vi "SetAttributeViBoolean_CP_Monitor_PS_Waveform.vi"(7 "AttributeValue (Off)":bool, 8 "error in (no error)":errorcluster {"code" format="%.0x"}, 9 "AttributeID":u32(ring)=1150049 items=["CHANNELPOWER_AVERAGE_ENABLED"=1150049, "CHANNELPOWER_DETECTOR_AUTO"=1150109, "CHANNELPOWER_DISPLAY_BAR_GRAPH_ENABLED"=1190232, "CHANNELPOWER_DISPLAY_WINDOWY_AUTO_SCALE_ENABLED"=1190236, "CHANNELPOWER_FILTER_ENABLED"=1190238, "CHANNELPOWER_FREQUENCY_PHASE_NOISE_OPTION_AUTO_ENABLED"=1190659, "CHANNELPOWER_IF_GAIN_AUTO_ENABLED"=1150041, "CHANNELPOWER_IF_GAIN"=1150038, "CHANNELPOWER_MARKER_COUPLE_ENABLED"=1190668, "CHANNELPOWER_MARKER_ENABLED"=1190253, "CHANNELPOWER_POWER_LIMIT_ENABLED"=1191767, "CHANNELPOWER_PSD_LIMIT_ENABLED"=1191690, "CHANNELPOWER_SWEEPCOUPLING_RESOLUTION_BANDWIDTH_AUTO_ENABLED"=1190257, "CHANNELPOWER_SWEEPCOUPLING_SWEEP_TIME_AUTO_ENABLED"=1190260, "CHANNELPOWER_SWEEPCOUPLING_VIDEO_BANDWIDTH_AUTO_ENABLED"=1190263, "CONTINUOUS_PEAK_SEARCH_ENABLED"=1191709, "MONITOR_AVERAGE_ENABLED"=1190349, "MONITOR_DISPLAY_AUTO_WINDOWY_SCALE_ENABLED"=1190354, "MONITOR_FREQUENCY_SPAN_RESOLUTION_BANDWIDTH_RATIO_AUTO_ENABLED"=1190345, "MONITOR_MARKER_COUPLE_ENABLED"=1190371, "MONITOR_MARKER_ENABLED"=1191684, "MONITOR_SWEEPCOUPLING_RESOLUTION_BANDWIDTH_AUTO_ENABLED"=1190361, "MONITOR_SWEEPCOUPLING_SWEEP_TIME_AUTO_ENABLED"=1190364, "MONITOR_SWEEPCOUPLING_VIDEO_BANDWIDTH_AUTO_ENABLED"=1190366, "MONITOR_SWEEPCOUPLING_VIDEO_BANDWIDTH_RATIO_AUTO_ENABLED"=1150113, "MONITOR_TRACE_DETECTOR_TYPE_AUTO_ENABLED"=1190347, "MONITOR_TRACE_DISPLAY_ENABLED"=1190009, "MONITOR_TRACE_UPDATE_ENABLED"=1190040, "POWER_STATISTICS_DISPLAY_GAUSSIAN_LINE_ENABLED"=1190431, "POWER_STATISTICS_DISPLAY_REFERENCE_TRACE_ENABLED"=1190432, "POWER_STATISTICS_IF_GAIN_AUTO_ENABLED"=1190419, "POWER_STATISTICS_IF_GAIN"=1190418, "POWER_STATISTICS_MARKER_COUPLE_ENABLED"=1190426, "POWER_STATISTICS_MARKER_ENABLED"=1191685, "WAVEFORM_ADC_DITHER_AUTO_ENABLED"=1190536, "WAVEFORM_ADC_DITHER_ENABLED"=1190535, "WAVEFORM_AVERAGE_ENABLED"=1190538, "WAVEFORM_AVERAGE_TIME_AVERAGE_COUNT_AUTO_ENABLED"=1191503, "WAVEFORM_DISPLAY_IQWAVEFORM_VIEW_WINDOWX_AUTO_SCALE_ENABLED"=1191577, "WAVEFORM_DISPLAY_IQWAVEFORM_VIEW_WINDOWY_AUTO_SCALE_ENABLED"=1191581, "WAVEFORM_DISPLAY_WINDOWX_AUTO_SCALE_ENABLED"=1190547, "WAVEFORM_DISPLAY_WINDOWY_AUTO_SCALE_ENABLED"=1190550, "WAVEFORM_FILTER_BANDWIDTH_AUTO_ENABLED"=1191499, "WAVEFORM_FREQUENCY_SYNTHESIS_STATE_AUTO_ENABLED"=1191507, "WAVEFORM_IF_GAIN_AUTO_ENABLED"=1190532, "WAVEFORM_MARKER_COUPLE_ENABLED"=1190554, "WAVEFORM_MARKER_ENABLED"=1190556], 10 "RepCapIdentifier":string, 11 "instrument handle":refnum<k15>) -> (0 "error out":errorcluster {"code" format="%.0x"}, 3 "instrument handle out":refnum<k15>)   [LabVIEW 2021, in "Keysight XSAnVMA.lvlib"]
doc: "Sets Boolean Attribute from instrumrnt driver.\nThe following attributes are supported:\n\nCHANNELPOWER_AVERAGE_ENABLED\nCHANNELPOWER_DETECTOR_AUTO\nCHANNELPOWER_DISPLAY_BAR_GRAPH_ENABLED\nCHANNELPOWER_DISPLAY_WINDOWY_AUTO_SCALE_ENABLED\nCHANNELPOWER_FILTER_ENABLED\nCHANNELPOWER_FREQUENCY_PHASE_NOISE_OPTION_AUTO_ENABLED\nCHANNELPOWER_IF_GAIN_AUTO_ENABLED\nCHANNELPOWER_IF_GAIN\nCHANNELPOWER_MARKER_COUPLE_ENABLED\nCHANNELPOWER_MARKER_ENABLED\nCHANNELPOWER_POWER_LIMIT_ENABLED\nCHANNELPOWER_PSD_LIMIT_ENABLED\nCHANNELPOWER_SWEEPCOUPLING_RESOLUTION_BANDWIDTH_AUTO_ENABLED\nCHANNELPOWER_SWEEPCOUPLING_SWEEP_TIME_AUTO_ENABLED\nCHANNELPOWER_SWEEPCOUPLING_VIDEO_BANDWIDTH_AUTO_ENABLED\nCONTINUOUS_PEAK_SEARCH_ENABLED\nMONITOR_AVERAGE_ENABLED\nMONITOR_DISPLAY_AUTO_WINDOWY_SCALE_ENABLED\nMONITOR_FREQUENCY_SPAN_RESOLUTION_BANDWIDTH_RATIO_AUTO_ENABLED\nMONITOR_MARKER_COUPLE_ENABLED\nMONITOR_MARKER_ENABLED\nMONITOR_SWEEPCOUPLING_RESOLUTION_BANDWIDTH_AUTO_ENABLED\nMONITOR_SWEEPCOUPLING_SWEEP_TIME_AUTO_ENABLED\nMONITOR_SWEEPCOUPLING_VIDEO_BANDWIDTH_AUTO_ENABLED\nMONITOR_SWEEPCOUPLING_VIDEO_BANDWIDTH_RATIO_AUTO_ENABLED\nMONITOR_TRACE_DETECTOR_TYPE_AUTO_ENABLED\nMONITOR_TRACE_DISPLAY_ENABLED\nMONITOR_TRACE_UPDATE_ENABLED\nPOWER_STATISTICS_DISPLAY_GAUSSIAN_LINE_ENABLED\nPOWER_STATISTICS_DISPLAY_REFERENCE_TRACE_ENABLED\nPOWER_STATISTICS_IF_GAIN_AUTO_ENABLED\nPOWER_STATISTICS_IF_GAIN\nPOWER_STATISTICS_MARKER_COUPLE_ENABLED\nPOWER_STATISTICS_MARKER_ENABLED\nWAVEFORM_ADC_DITHER_AUTO_ENABLED\nWAVEFORM_ADC_DITHER_ENABLED\nWAVEFORM_AVERAGE_ENABLED\nWAVEFORM_AVERAGE_TIME_AVERAGE_COUNT_AUTO_ENABLED\nWAVEFORM_DISPLAY_IQWAVEFORM_VIEW_WINDOWX_AUTO_SCALE_ENABLED\nWAVEFORM_DISPLAY_IQWAVEFORM_VIEW_WINDOWY_AUTO_SCALE_ENABLED\nWAVEFORM_DISPLAY_WINDOWX_AUTO_SCALE_ENABLED\nWAVEFORM_DISPLAY_WINDOWY_AUTO_SCALE_ENABLED\nWAVEFORM_FILTER_BANDWIDTH_AUTO_ENABLED\nWAVEFORM_FREQUENCY_SYNTHESIS_STATE_AUTO_ENABLED\nWAVEFORM_IF_GAIN_AUTO_ENABLED\nWAVEFORM_MARKER_COUPLE_ENABLED\nWAVEFORM_MARKER_ENABLED"
uses:
  <instrlib>/Keysight XSAnVMA/Keysight XSAnVMA.lvlib
  KtXSAnVMA_64.dll
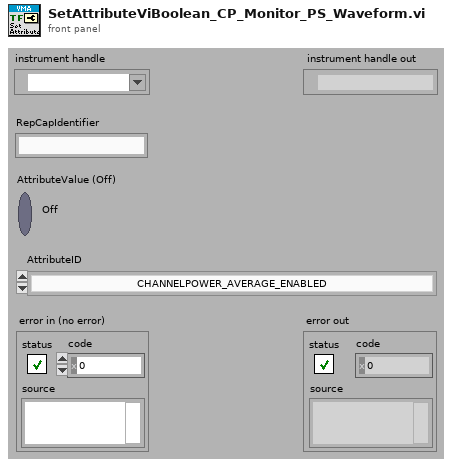
[diagram p1: front panel]
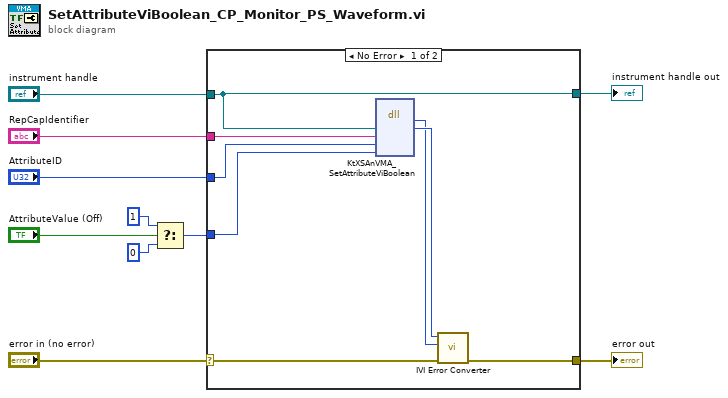
[diagram p0: block diagram]
diagram:
  n1 = Select(t=u16 1, s="AttributeValue (Off)", f=u16 0) -> (s? t:f=w3:u16)
  n2 = case shown="No Error" "error in (no error)" {
    selector: "error in (no error)" -> [w16 w20]
    tunnel: [w15 w20] -> w10
    tunnel: "instrument handle" -> [w11 w19]
    tunnel: "RepCapIdentifier" -> [w14 _]
    tunnel: "AttributeID" -> [w13 _]
    tunnel: w3 -> [w12 _]
    tunnel: [w11 w19] -> w1
    frame No Error {
      n3 = dll-call lib="KtXSAnVMA**.dll" fn="KtXSAnVMA_SetAttributeViBoolean"("Vi"=w11, "RepCapIdentifier"=w14, "AttributeID"=w13, "AttributeValue"=w12) -> ("return type"=w17:i32, "Vi"=w18:u32)  [unwired: 6 in, 2 out]
      n4 = call <instrlib>:"IVI Error Converter.vi"("error in (no error)"=w16, "IVI error code (0)"=w17, "instrument handle"=w18) -> ("error out"=w15:errorcluster)  [unwired: 7 in, 1 out]
    }
    frame Error {
    }
  }
  "error out" <- w10
  "instrument handle out" <- w1
